vi "example_Job_Static_VI_Reference.vi"() -> ()   [LabVIEW 2013, in "openCronJob.lvlib" / "Job.StaticVIRef.lvclass"]
uses:
  Job.StaticVIRef.lvclass
  Job/Job.lvclass
  Job/Job.lvclass/Job.ctl
  Job/Read Abort Notifier.vi
panel:
  out "Job out":refnum<class "Job.lvclass">
  out "error out":errorcluster
  in  "Job":refnum<class "Job.lvclass">
  out "stdout":string
  in  "stdin":string
  # "Terminals can be anywhere on the front panel, and do not need to be connected to the ConPane"
  # "All terminals are optional, but:\n-- \"Job\" class input allows to monitor the Abort notifications from scheduler.\n-- \"Job\" class output allows to insert key-value pairs into data map.\n-- stdin allows to pass in commands into the job\n-- stdout allows to send back a response to the scheduler after execution completes\n-- error output terminal returns the exception code to the scheduler\n-- stdin and stdout are \"named\" and must be configured with the Static VI refnum,\nunless they take the default stdin and stdout values, in which case they will be found\nnonetheless."
  # "Can be more\nspecific than\nbase class, but\nmust thrall input\notherwise async\nmight ignore."
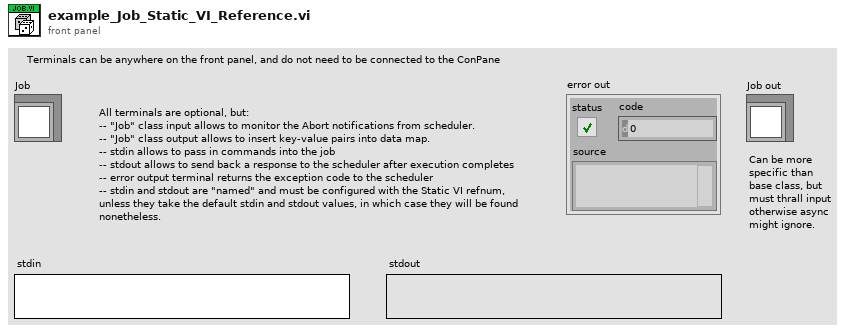
[diagram p1: front panel]
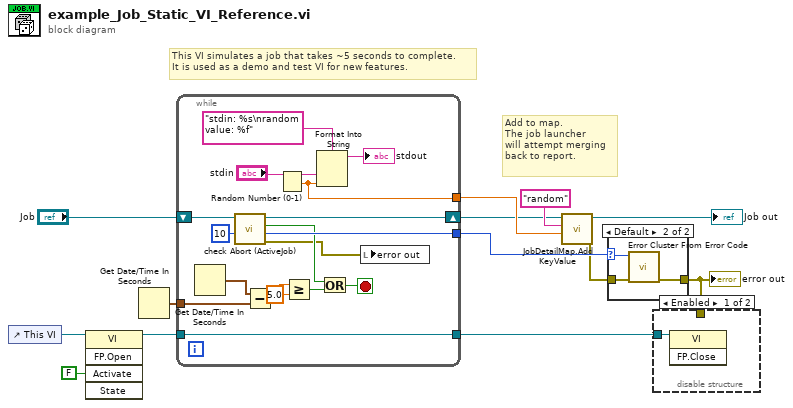
[diagram p0: block diagram]
diagram:
  # "Add to map.\nThe job launcher\nwill attempt merging\nback to report."
  # "This VI simulates a job that takes ~5 seconds to complete.\nIt is used as a demo and test VI for new features."
  n1 = control-ref of="This VI"() -> (w8:refnum<vi>)
  n2 = invoke class="VI" method="FP.Open"(reference=w8, "Activate"=FALSE ("Activate?")) -> (reference out=w13:refnum<vi>)  [unwired: 3 in, 4 out]
  n3 = Get Date/Time In Seconds() -> (seconds since 1Jan1904=w6:timestamp)
  n4 = while {
    tunnel: w6 -> [w30]
    tunnel: [w22] -> w11
    tunnel: [w20] -> w10
    tunnel: w13 -> [w17]
    tunnel: [w17] -> w12
    shift-right: [w15] -> w3
    shift-left: "Job" -> [w24]
    stop <- w26 stop-if-true
    n5 = Get Date/Time In Seconds() -> (seconds since 1Jan1904=w18:timestamp)
    n6 = call "check Abort (ActiveJob).vi"("timeout (0 ms)"=10 ("timeout in ms (-1)"), "Job in"=w24) -> ("error out"=w14:errorcluster, "exception"=w22:i32, "Abort"=w16:bool, "Job out"=w15:refnum<class "Job.lvclass">)  [unwired: 6 in]
    n7 = Subtract(x=w18, y=w30) -> (x-y=w29:dbl)
    n8 = Random Number (0-1)() -> (number: 0 to 1=w20:dbl)
    n9 = Greater Or Equal?(x=w29, y=5.0) -> (x >= y?=w27:bool)
    n10 = Format Into String(format string="stdin: %s\nrandom value: %f", "stdin", w20) -> (resulting string=→"stdout":string)  [unwired: 2 in, 1 out]
    n11 = Or(x=w16, y=w27) -> (x .or. y?=w26:bool)
    n12 = local write "error out"(w14) -> ()
  }
  n13 = call "JobDetailMap.Add KeyValue.vi"("Value"=w10, "Key"="random", "Job in"=w3) -> ("error out"=w2:errorcluster, "Job out"=→"Job out":refnum<class "Job.lvclass">)  [unwired: 7 in]
  n14 = case shown="Default" w11 {
    selector: w11 -> [_ w34]
    tunnel: [w31 w33] -> w1
    tunnel: w2 -> [w31 w32]
    frame 0 {
    }
    frame Default {
      n15 = call <vilib>:"Error Cluster From Error Code.vi"("error in (no error)"=w32, "error code (0)"=w34) -> ("error out"=w33:errorcluster)  [unwired: 7 in]
    }
  }
  "error out" <- w1
  n16 = disable-structure shown="Enabled" {
    disable-tunnel: w12 -> [w35 _]
    disable-tunnel: w1 -> [_ _]
    frame Enabled {
      n17 = invoke class="VI" method="FP.Close"(reference=w35) -> ()  [unwired: 2 in, 3 out]
    }
    frame Disabled {
    }
  }
